vi "CtrlTreeSelectionAsStringArray.vi"(8 "error in (no error)":errorcluster, 11 "TreeControl in":refnum<vi>) -> (0 "error out":errorcluster, 2 "Selection":string[](array[string]), 3 "TreeControl out":refnum<vi>)   [LabVIEW 2021]
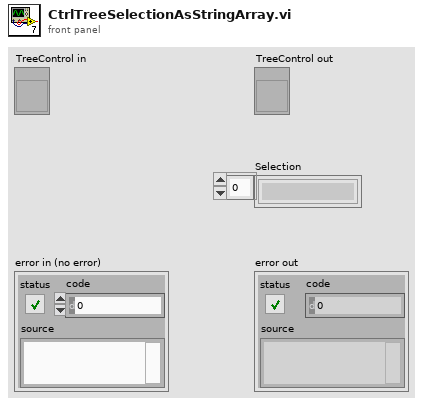
[diagram p1: front panel]
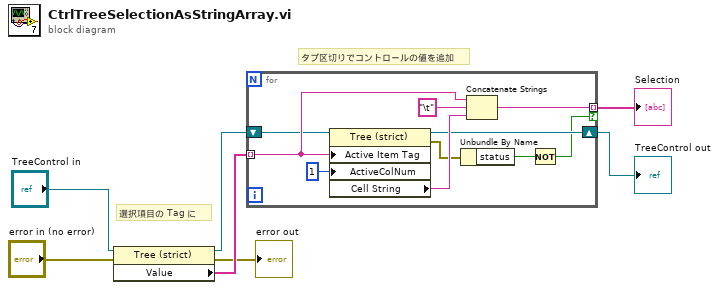
[diagram p0: block diagram]
diagram:
  # "選択項目の Tag に"
  # "タブ区切りでコントロールの値を追加"
  n1 = property class="Tree (strict)"(reference="TreeControl in", error in="error in (no error)") -> (reference out=w6:refnum<vi>, error out=→"error out":errorcluster, "Value"=w5:string[])
  n2 = for {
    tunnel: w5 -> [w15] mode=indexing
    shift-right: [w13] -> w7
    shift-left: w6 -> [w14]
    tunnel: [w12] -> w1 mode=indexing if=w8
    n3 = property class="Tree (strict)"(reference=w14, "Active Item Tag"=w15, "ActiveColNum"=1 ("Active Cell:Active Column Number")) -> (reference out=w13:refnum<vi>, error out=w10:errorcluster, "Cell String"=w16:string)  [unwired: 1 in]
    n4 = Unbundle By Name(w10) -> ("status"=w9:bool)
    n5 = Concatenate Strings(w15, "\t" ("string"), w16) -> (w12:string)
    n6 = Not(x=w9) -> (.not. x?=w8:bool)
  }
  "Selection" <- w1
  "TreeControl out" <- w7
